vi "Scalar JSON text to Variant.vi"(6 "Type Enum":T1, 8 "error in (no error)":errorcluster, 9 "Variant (Data Type)":variant, 10 "Offset":i32, 11 "JSON":string) -> (0 "error out":errorcluster, 1 "Variant out":variant)   [LabVIEW 2013, in "JSONtext.lvlib"]
uses:
  JSONtext.lvlib
  <vilib>/Utility/VariantDataType/Type.ctl
  Advance past String.vi
  String Subset.vi
  support/Strip Quotes and Unescape.vi
  Get Number Text (inlined).vi
  Advance past Number.vi
  Parsing Error.vi
  support/Unescape JSON string.vi
  <vilib>/Utility/VariantDataType/VariantType.lvlib
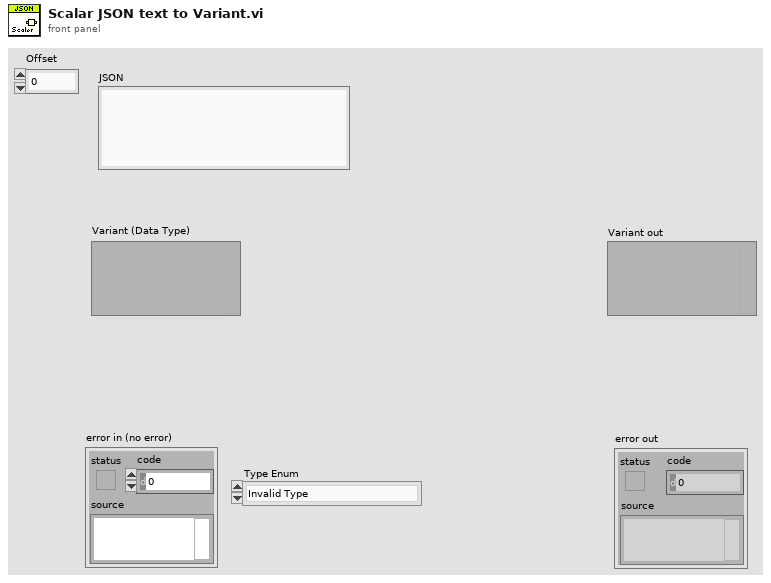
[diagram p1: front panel]
types:
  T1 = typedef "VariantType.lvlib/Type.ctl" = enum8{"Invalid Type", "Void", "I8", "I16", "I32", "I64", "U8", "U16", "U32", "U64", "Single Float", "Double Float", "Extended Float", "Single Complex", "Double Complex", "Extended Complex", "Enum U8", "Enum U16", "Enum U32", "Enum U64", "Single Float With Unit", "Double Float With Unit", "Extended Float With Unit", "Single Complex with Unit", "Double Complex with Unit", "Extended Complex with Unit", "Boolean", "String", "Path", "Picture", "Tag", "Array", "Cluster", "Variant", "LV Variant", "Waveform", "Timestamp", "Digital Waveform", "Digital Data", "ExpressData", "Refnum", "External Data", "VI", "Poly VI", "LabVIEW Class Instance", "Fixed Point"}
  T2 = typedef "JSONtext.lvlib/JSON Value Search.ctl" = enum16{"Parser Error", "In Object", "In Array", "String", "Number", "Leading Whitespace", "Object end", "Array end", "Value end", "Undefined"}
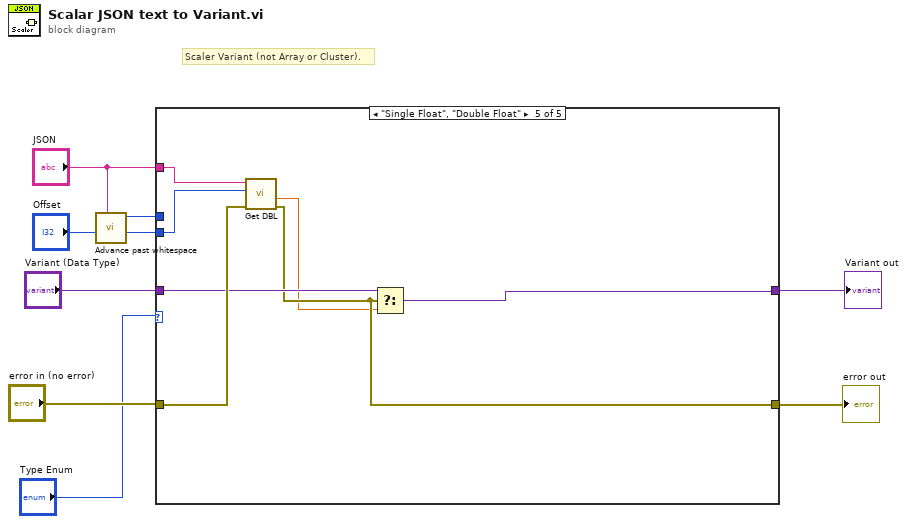
[diagram p0: block diagram]
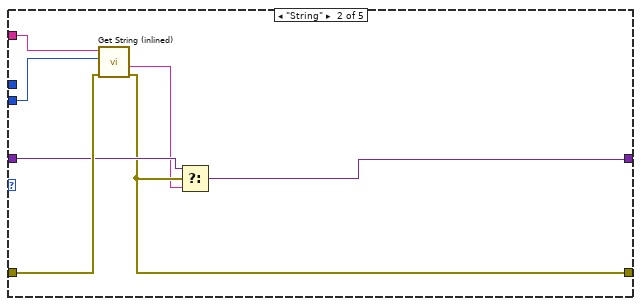
[diagram p3: hidden frame]
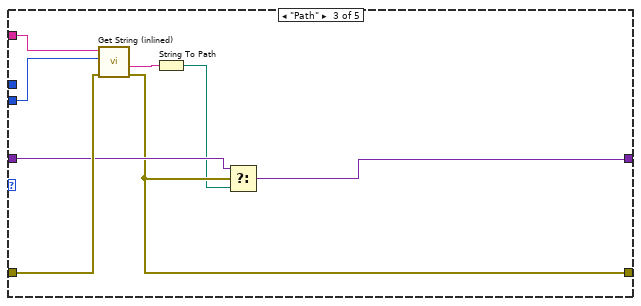
[diagram p4: hidden frame]
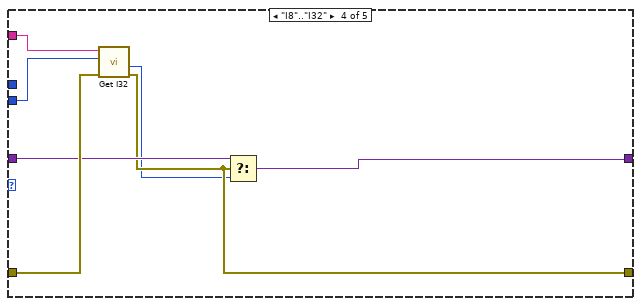
[diagram p5: hidden frame]
diagram:
  # "Scaler Variant (not Array or Cluster)."
  n1 = call "Advance past whitespace.vi"("JSON"="JSON", "Offset"="Offset") -> ("Offset past match"=w5:i32, "State"=w3:T2)  [unwired: 7 in, 1 out]
  n2 = case shown="\"Single Float\", \"Double Float\"" "Type Enum" {
    tunnel: "Variant (Data Type)" -> [w10 w15 w23 w31 w38]
    tunnel: "JSON" -> [_ w17 w25 w28 w35]
    tunnel: [w11 w13 w21 w29 w36] -> w8
    tunnel: "error in (no error)" -> [w11 w16 w24 w32 w39]
    tunnel: w5 -> [_ w18 w26 w33 w40]
    tunnel: [w10 w14 w22 w30 w37] -> w7
    tunnel: w3 -> [_ _ _ _ _]
    frame "Invalid Type", Default {
    }
    frame "String" {
      n3 = call "Get String (inlined).vi"("error in (no error)"=w16, "Offset"=w18, "JSON"=w17) -> ("error out"=w13:errorcluster, "String"=w12:string)  [unwired: 7 in]
      n4 = Select(t=w15, s=w13, f=w12) -> (s? t:f=w14:variant)
    }
    frame "Path" {
      n5 = call "Get String (inlined).vi"("error in (no error)"=w24, "Offset"=w26, "JSON"=w25) -> ("error out"=w21:errorcluster, "String"=w19:string)  [unwired: 7 in]
      n6 = String To Path(string=w19) -> (path=w20:path)
      n7 = Select(t=w23, s=w21, f=w20) -> (s? t:f=w22:variant)
    }
    frame "I8".."I32" {
      n8 = call "Get I32.vi"("error in (no error)"=w32, "Offset"=w33, "JSON"=w28) -> ("error out"=w29:errorcluster, "Number"=w27:i32)  [unwired: 7 in]
      n9 = Select(t=w31, s=w29, f=w27) -> (s? t:f=w30:variant)
    }
    frame "Single Float", "Double Float" {
      n10 = call "Get DBL.vi"("error in (no error)"=w39, "Offset"=w40, "JSON"=w35) -> ("error out"=w36:errorcluster, "Number"=w34:dbl)  [unwired: 7 in]
      n11 = Select(t=w38, s=w36, f=w34) -> (s? t:f=w37:variant)
    }
  }
  "Variant out" <- w7
  "error out" <- w8
